vi "HistStat(SubVI).vi"(2 "Binary Image":T1, 3 "Original Image":T1) -> (0 "HistStat":dbl[](array[numeric]), 1 "Gray Image":T1(plugin-control))   [LabVIEW 2015]
uses:
  <vilib>/vision/Image Controls.llb/IMAQ Image.ctl
  <vilib>/vision/NI_Vision_Development_Module.lvlib
  2-top_features_oilseed/HistProperty.dll
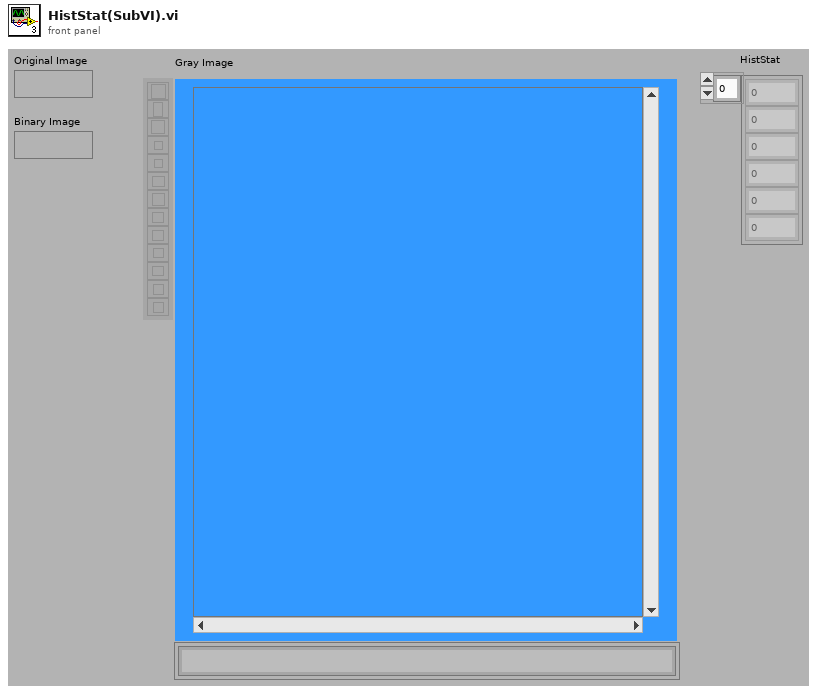
[diagram p1: front panel]
types:
  T1 = typedef "IMAQ Image.ctl" = refnum<image>
  T2 = typedef "Image Type" = u32
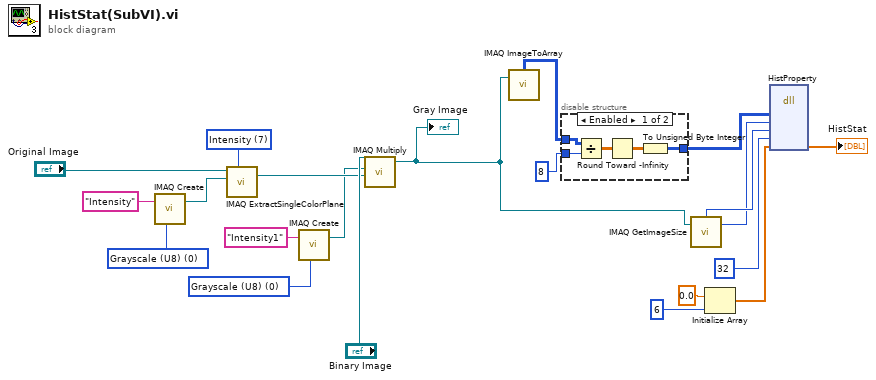
[diagram p0: block diagram]
diagram:
  w5 = T2 0 items=["Grayscale (U8)", "Grayscale (I16)", "Grayscale (SGL)", "Complex (CSG)", "RGB (U32)", "HSL (U32)", "RGB (U64)", "Grayscale (U16)"] ("Image Type")
  w2 = T2 0 items=["Grayscale (U8)", "Grayscale (I16)", "Grayscale (SGL)", "Complex (CSG)", "RGB (U32)", "HSL (U32)", "RGB (U64)", "Grayscale (U16)"] ("Image Type")
  w1 = 7 items=["Red", "Green", "Blue", "Hue", "Saturation", "Luminance", "Value", "Intensity"] ("Color Plane")
  n1 = call "IMAQ Create"("Image Name"="Intensity", "Image Type"=w2) -> ("New Image"=w9:T1)  [unwired: 2 in, 2 out]
  n2 = call "IMAQ ExtractSingleColorPlane"("Color Plane"=w1, "Image Dst"=w9, "Image Src"="Original Image") -> ("Image Dst Out"=w7:T1)  [unwired: 1 in, 7 out]
  n3 = call "IMAQ Create"("Image Name"="Intensity1", "Image Type"=w5) -> ("New Image"=w6:T1)  [unwired: 2 in, 2 out]
  n4 = call "IMAQ Multiply"("Image Src A"="Binary Image", "Image Dst"=w6, "Image Src B"=w7) -> ("Image Dst Out"=w21:T1)  [unwired: 2 in, 3 out]
  "Gray Image" <- w21
  n5 = call "IMAQ ImageToArray"("Image"=w21) -> ("Image Pixels (U8)"=w11:u8[][])  [unwired: 2 in, 5 out]
  n6 = disable-structure shown="Enabled" {
    disable-tunnel: w11 -> [w26 w27]
    disable-tunnel: u8 8 ("y") -> [w25 _]
    disable-tunnel: [w22 w27] -> w13
    frame Enabled {
      n7 = Divide(x=w26, y=w25) -> (x/y=w24:dbl[][])
      n8 = Round Toward -Infinity(1:w24) -> (0:w23:dbl[][])
      n9 = To Unsigned Byte Integer(number=w23) -> (unsigned 8bit integer=w22:u8[][])
    }
    frame Disabled {
    }
  }
  n10 = call "IMAQ GetImageSize"("Image"=w21) -> ("Y Resolution"=w14:i32, "X Resolution"=w15:i32)  [unwired: 1 in, 3 out]
  n11 = Initialize Array(0.0 ("element"), 6 ("dimension size")) -> (w18:dbl[])
  n12 = dll-call lib="H:/2-top_features_oilseed/HistProperty.dll" fn="HistProperty"("Im"=w13, "row"=w14, "col"=w15, "G"=32, "HistStat"=w18) -> ("HistStat"=→"HistStat":dbl[])  [unwired: 7 in, 3 out]
